vi "Simulated Beam Response.vi"() -> ()   [LabVIEW 2011, in "Simulated Beam VIs.lvlib"]
uses:
  Simulated Beam VIs.lvlib
panel:
  in  "Simulated Beam Response":dbl[][](array[numeric])
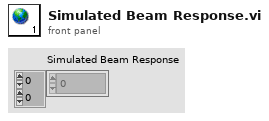
[diagram p1: front panel]
diagram:
